vi "Configure Route.vi"   [LabVIEW 2016, in "Keithley 2000.lvlib"]
doc: "This VI controls the switch functionality of an internal or external scanner card. It can be used to open or close one or more channels.\n\nNote:\nThis is a polymorphic VI. You can wire a single channel number or an array of channel numbers to configure multiple channels at once."
uses:
  Keithley 2000.lvlib
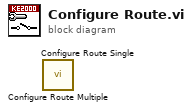
[diagram p0: block diagram]
diagram:
  n1 = call "Configure Route Multiple.vi"() -> ()  [unwired: 18 in, 2 out]
  n2 = call "Configure Route Single.vi"() -> ()  [unwired: 18 in, 2 out]
